vi "ContMeta.vi"(4 "Aux graph ref":refnum<vi>, 6 "CtrlRefsin":T3, 7 "slider refs in":T4, 9 "File Paths":T5={"Local Save Path"=path "\\\\smbhome.uscs.susx.ac.uk\\cv222/Desktop/data", "Newton Save Path"=path "Z:/#Projects/Entanglement/data", "File Name"="test", "LocalSave"=TRUE}, 10 "Compiler Settings":T6={"Python Path"=path "", "Main File"="makesequence.py", "Meta File"="makesequence.py", "Aux File"="makesequence.py", "Pre File"="metascript.txt"}, 11 "ControllerSettingsRef":refnum<vi>) -> ()   [LabVIEW 2019]
uses:
  PulseCompiler/CompilerSettings.ctl
  controls/FilePaths.ctl
  controls/FluoSettings.ctl
  controls/xAOMSettings/XAOMsetting.xctl
  controls/PowerStableSettings.ctl
  PulseControl.ctl
  Compiler/Params.ctl
  controls/ControllerSettings.ctl
  controls/GlobalExp.vi
  Global.lvlib
panel:
  out "calib":bool
  out "Aux Pulse":T1
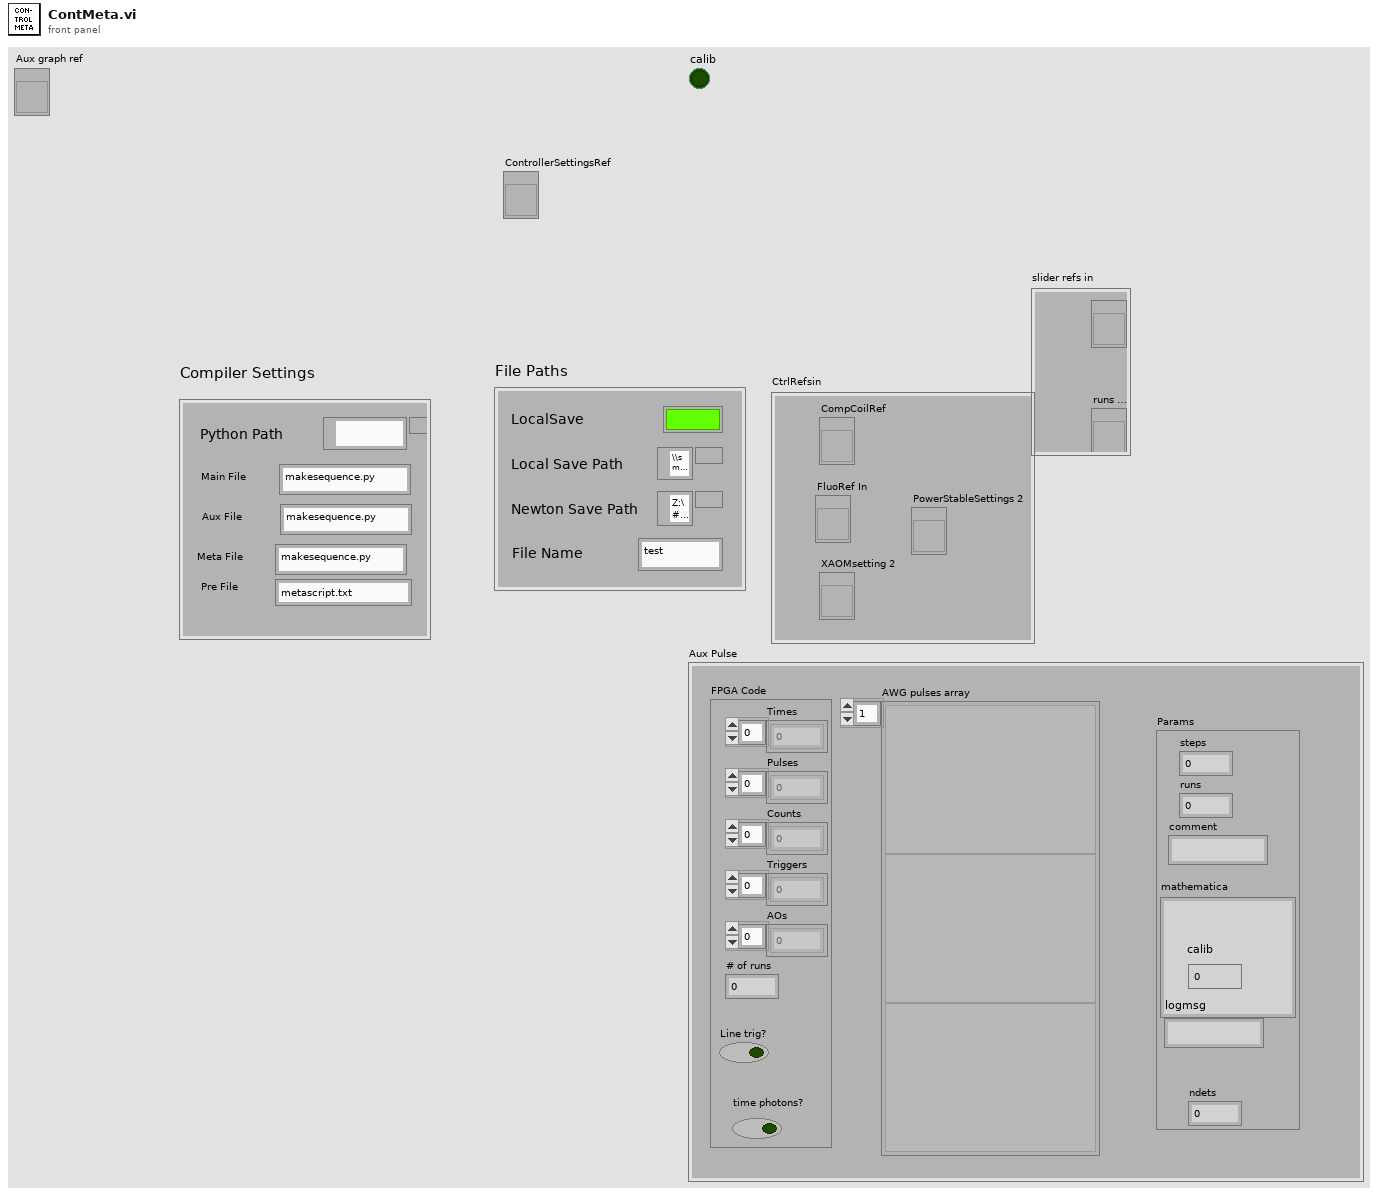
[diagram p1: front panel]
types:
  T1 = typedef "PulseControl.ctl" = cluster{"FPGA Code":cluster{"Times":u32[], "Pulses":u64[], "Counts":u8[], "Triggers":u8[], "AOs":u8[], "# of runs":i32, "Line trig?":bool, "time photons?":bool}, "AWG pulses array":variant[], "Params":T2}
  T2 = typedef "Params.ctl" = cluster{"steps":i16, "runs":i16, "comment":string, "mathematica":string, "calib":i8, "logmsg":string, "ndets":i16}
  T3 = cluster{"CompCoilRef":refnum<vi>, "FluoRef In":refnum<vi>, "XAOMsetting 2":refnum<vi>, "PowerStableSettings 2":refnum<vi>}
  T4 = cluster{"steps slider ref":refnum<vi>, "runs slider ref":refnum<vi>}
  T5 = typedef "FilePaths.ctl" = cluster{"Local Save Path":path, "Newton Save Path":path, "File Name":string, "LocalSave":bool}
  T6 = typedef "CompilerSettings.ctl" = cluster{"Python Path":path, "Main File":string, "Meta File":string, "Aux File":string, "Pre File":string}
  T7 = enum16{"Innit", "Stop", "Idle", "MainRunning", "AuxRunning"}
  T8 = typedef "MasterExpControl.ctl" = cluster{"Main Steps":dbl, "Main Runs":dbl, "ExpStatus":enum16{"Innit", "Stop", "Idle", "MainRunning", "AuxRunning"}, "Main Current Step":dbl, "ExpNum":dbl, "NewData":bool, "date":string, "command":string, "Stop":bool, "Pause":bool, "Mathematica":string, "Main/Meta":bool, "UpdateMath":bool, "Camera":bool, "MetaExpOver":bool, "NextMetaExp":bool}
  T9 = typedef "ControllerSettings.ctl" = cluster{"Aux Sequence":bool, "Camera":bool, "Recrystallize":bool, "Raw graph":bool, "Mean graph":bool, "Calculate probs":bool, "Find fit":bool, "ReX Time [s] :":dbl, "Lock Voltage :":dbl, "Line trig ":bool, "Check Fluo":bool, "Pre Sequence":bool}
  T10 = cluster{"readout":u32[][], "kinetic series data":i32[][][][], "camera dim":cluster{i32, i32, i32, i32}}
  T11 = cluster{"readout out 2":dbl[][], "kinetic series data":i32[][][][], "camera dim":cluster{i32, i32, i32, i32}}
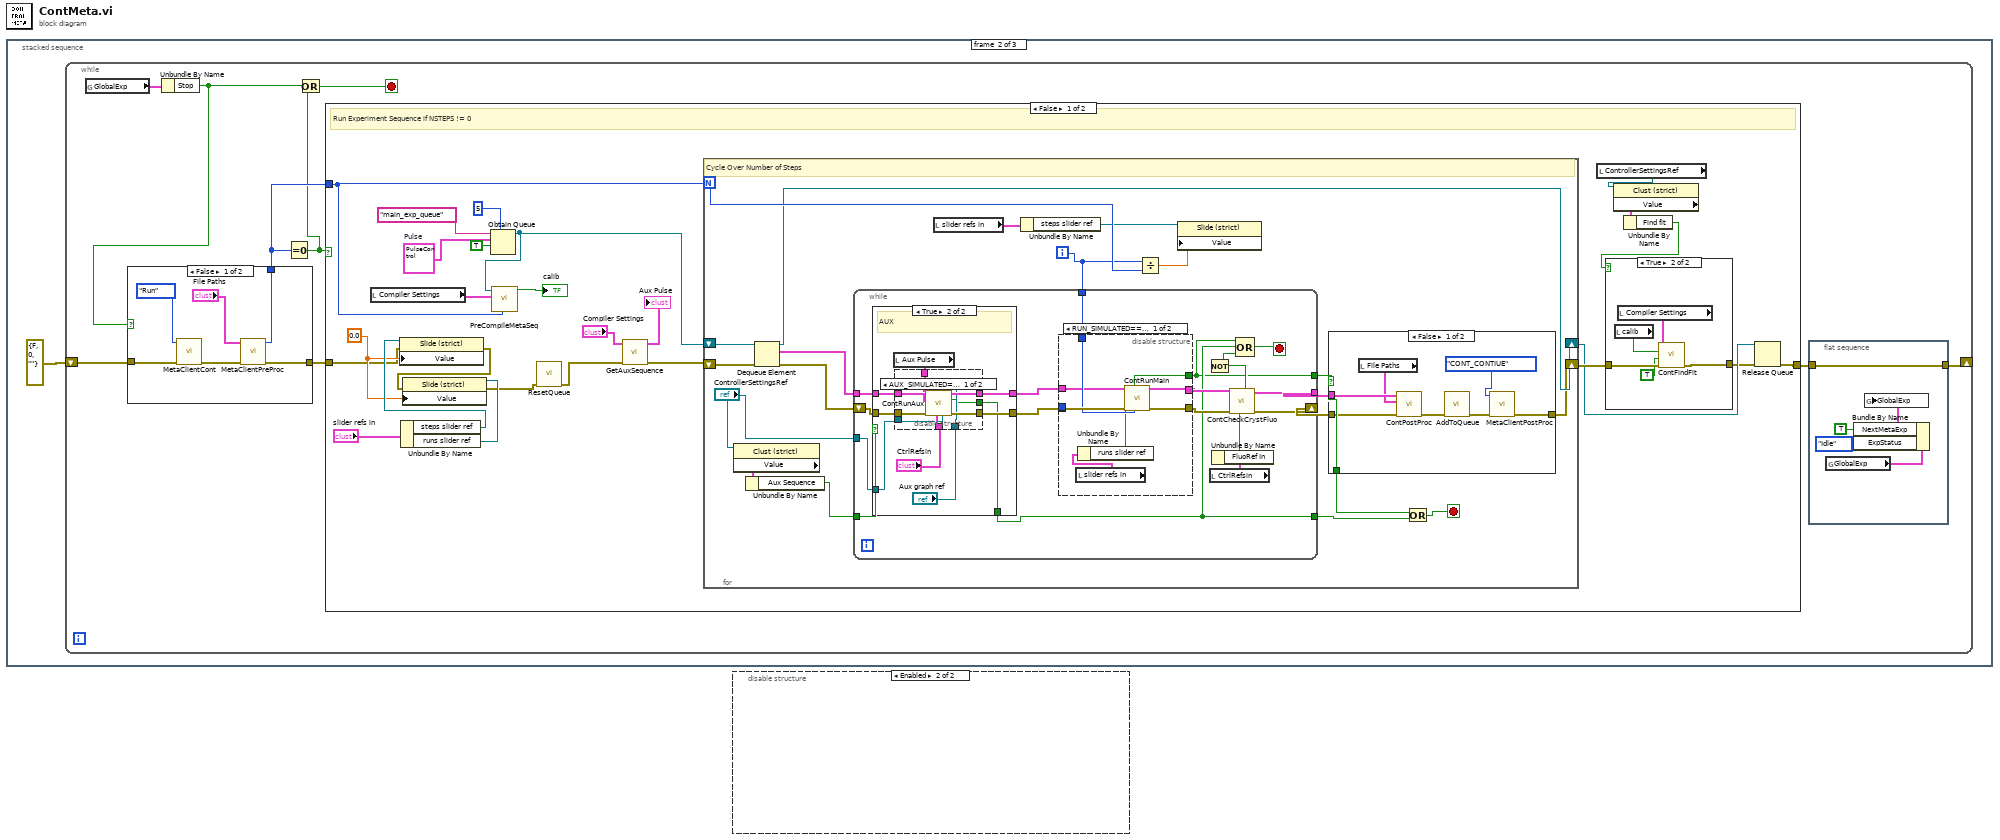
[diagram p0: block diagram]
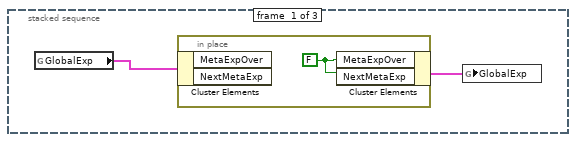
[diagram p2: hidden frame]
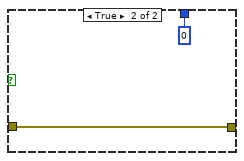
[diagram p3: hidden frame]
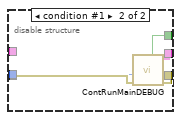
[diagram p5: hidden frame]
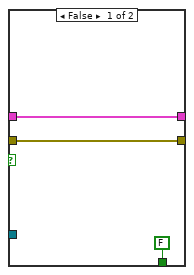
[diagram p6: hidden frame]
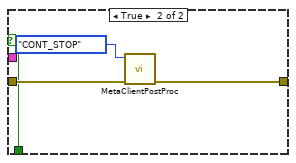
[diagram p8: hidden frame]
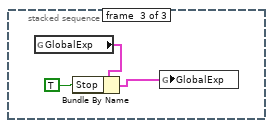
[diagram p10: hidden frame]
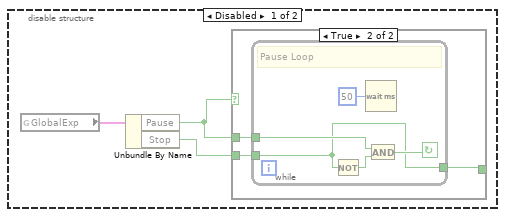
[diagram p11: hidden frame]
diagram:
  n1 = stacked-sequence {
    frame #0 {
      n2 = global read "GlobalExp.vi" "GlobalExp"() -> (w2:T8)
      n3 = in-place {
        w3 = FALSE
        n4 = in-place-cluster #1(w2) -> ()  [unwired: 2 out]
        n5 = in-place-cluster #1("MetaExpOver"=w3, "NextMetaExp"=w3) -> (w1:T8)
      }
      n6 = global write "GlobalExp.vi" "GlobalExp"(w1) -> ()
    }
    frame #1 {
      n7 = while {
        shift-right: [w11] -> _
        shift-left: errorcluster {"status"=FALSE, "code"=0, "source"=""} ("error out") -> [w13]
        stop <- w9 stop-if-true
        n8 = global read "GlobalExp.vi" "GlobalExp"() -> (w6:T8)
        n9 = Unbundle By Name(w6) -> ("Stop"=w8:bool)
        n10 = case shown="False" w8 {
          tunnel: w13 -> [w19 w20]
          tunnel: [w15 w20] -> w12
          tunnel: [w14 0 ("steps")] -> w10
          frame False {
            n11 = call "MetaClientCont.vi"("error in (no error)"=w19, "Action"=enum16{"Run", "Exit"}."Run") -> ("error out"=w17:errorcluster)  [unwired: 8 in, 1 out]
            n12 = call "MetaClientPreProc.vi"("error in (no error)"=w17, "File Paths"="File Paths") -> ("error out"=w15:errorcluster, "steps"=w14:i32)  [unwired: 7 in, 1 out]
          }
          frame True {
          }
        }
        n13 = Equal To 0?(x=w10) -> (x = 0?=w7:bool)
        n14 = Or(x=w8, y=w7) -> (x .or. y?=w9:bool)
        n15 = case shown="False" w7 {
          tunnel: w12 -> [w31 w140]
          tunnel: [w23 w140] -> w5
          tunnel: w10 -> [w36 _]
          frame False {
            w32 = 0.0 ("Value")
            w43 = T1 {"FPGA Code"={"Times"=[], "Pulses"=[], "Counts"=[], "Triggers"=[], "AOs"=[], "# of runs"=0, "Line trig?"=FALSE, "time photons?"=FALSE}, "AWG pulses array"=[], "Params"={"steps"=0, "runs"=0, "comment"="", "mathematica"="", "calib"=0, "logmsg"="", "ndets"=0}}  # Pulse
            # "Run Experiment Sequence if NSTEPS != 0"
            n16 = local read "Compiler Settings"() -> (w41:T6)
            n17 = Unbundle By Name("slider refs in") -> ("steps slider ref"=w33:refnum<vi>, "runs slider ref"=w34:refnum<vi>)
            n18 = property class="Slide (strict)"(reference=w33, error in=w31, "Value"=w32) -> (error out=w30:errorcluster)  [unwired: 1 out]
            n19 = property class="Slide (strict)"(reference=w34, error in=w30, "Value"=w32) -> (error out=w28:errorcluster)  [unwired: 1 out]
            n20 = Obtain Queue(max queue size (-1, unlimited)=5, name (unnamed)="main_exp_queue", element data type=w43, create if not found? (T)=TRUE) -> (queue out=w40:refnum<queue>)  [unwired: 1 in, 2 out]
            n21 = call "PreCompileMetaSeq.vi"("steps"=w36, "Compiler Settings"=w41, "queue in"=w40) -> ("calib"=→"calib":bool)  [unwired: 7 in, 1 out]
            n22 = call "ResetQueue.vi"("error constant"=w28) -> ("error constant 2"=w29:errorcluster)  [unwired: 10 in]
            n23 = call "GetAuxSequence.vi"("error in (no error)"=w29, "Compiler Settings"="Compiler Settings") -> ("error out"=w47:errorcluster, "Aux Pulse"=→"Aux Pulse":T1)  [unwired: 8 in]
            n24 = for {
              N: w36 -> [w71]
              shift-right: [w59] -> w38
              shift-left: w47 -> [w68]
              shift-right: [w60] -> w25
              shift-left: w40 -> [w66]
              i -> [w61]
              stop <- w58 stop-if-true
              # "Cycle Over Number of Steps"
              n25 = property class="Clust (strict)"(reference="ControllerSettingsRef") -> ("Value"=w55:T9)  [unwired: 1 in, 2 out]
              n26 = Unbundle By Name(w55) -> ("Aux Sequence"=w64:bool)
              n27 = Dequeue Element(queue=w66, error in (no error)=w68) -> (queue out=w60:refnum<queue>, element=w65:T1, error out=w67:errorcluster)  [unwired: 1 in, 1 out]
              n28 = while {
                tunnel: [w75] -> w72
                tunnel: w65 -> [w90]
                tunnel: [w83] -> w62
                tunnel: w61 -> [w87]
                tunnel: "ControllerSettingsRef" -> [w85]
                shift-right: [w82] -> w63
                shift-left: w67 -> [w91]
                tunnel: w64 -> [w88]
                tunnel: [w76] -> w56
                stop <- w74 stop-if-true
                n29 = case shown="True" w88 {
                  tunnel: [w107 w117] -> w86
                  tunnel: w91 -> [w108 w116]
                  tunnel: [w108 w115] -> w89
                  tunnel: w90 -> [w107 w112]
                  tunnel: [FALSE ("Aux stopped") w110] -> w76
                  tunnel: w85 -> [_ w109]
                  frame False {
                  }
                  frame True {
                    # "AUX"
                    n30 = local read "Aux Pulse"() -> (w111:T1)
                    n31 = disable-structure shown="AUX_SIMULATED==FALSE, Default" {
                      disable-tunnel: [w126 _] -> w117
                      disable-tunnel: w116 -> [w125 w127]
                      disable-tunnel: [w124 w127] -> w115
                      disable-tunnel: "Aux graph ref" -> [w123 _]
                      disable-tunnel: "CtrlRefsin" -> [w122 _]
                      disable-tunnel: w112 -> [w121 _]
                      disable-tunnel: w111 -> [w120 _]
                      disable-tunnel: [w119 _] -> w110
                      disable-tunnel: w109 -> [w118 _]
                      frame condition #0 (active) {
                        n32 = call "ContRunAux.vi"("ControllerSettingsRef"=w118, "CtrlRefsin"=w122, "Aux chart ref in"=w123, "error in (no error)"=w125, "Aux pulse in"=w120, "Main Pulse In"=w121) -> ("error out"=w124:errorcluster, "Aux stopped"=w119:bool, "Main Pulse Out"=w126:T1)  [unwired: 3 in]
                      }
                      frame condition #1 {
                      }
                    }
                  }
                }
                n33 = disable-structure shown="RUN_SIMULATED==FALSE" {
                  disable-tunnel: [w97 w105] -> w84
                  disable-tunnel: w89 -> [w99 w104]
                  disable-tunnel: [w98 w103] -> w81
                  disable-tunnel: [w96 w101] -> w75
                  disable-tunnel: _ -> [_ w100]
                  disable-tunnel: w87 -> [w95 _]
                  disable-tunnel: w86 -> [w92 _]
                  frame condition #0 (active) {
                    n34 = local read "slider refs in"() -> (w94:T4)
                    n35 = Unbundle By Name(w94) -> ("runs slider ref"=w93:refnum<vi>)
                    n36 = call "ContRunMain.vi"("Step Number"=w95, "error in"=w99, "runs slider ref"=w93, "Main Pulse In"=w92) -> ("error out"=w98:errorcluster, "readout"=w97:T10, "Stop"=w96:bool)  [unwired: 5 in]
                  }
                  frame condition #1 {
                    n37 = call "ContRunMainDEBUG.vi"("error in (no error)"=w104, "step num"=w100) -> ("error out"=w103:errorcluster, "readout"=w105:T11, "Stop"=w101:bool, "runs slider ref"=w102:refnum<vi>)  [unwired: 6 in]
                  }
                }
                n38 = local read "CtrlRefsin"() -> (w78:T3)
                n39 = Unbundle By Name(w78) -> ("FluoRef In"=w77:refnum<vi>)
                n40 = call "ContCheckCrystFluo.vi"("FluoRef In"=w77, "error in (no error)"=w81, "readout"=w84) -> ("error out"=w82:errorcluster, "readout 2"=w83:T10, "restart step?"=w79:bool)  [unwired: 6 in]
                n41 = Not(x=w79) -> (.not. x?=w80:bool)
                n42 = Compound Arithmetic op=OR(w75, w76, w80) -> (w74:bool)
              }
              n43 = local read "slider refs in"() -> (w70:T4)
              n44 = Unbundle By Name(w70) -> ("steps slider ref"=w69:refnum<vi>)
              n45 = Divide(x=w61, y=w71) -> (x/y=w73:dbl)
              n46 = property class="Slide (strict)"(reference=w69, "Value"=w73) -> ()  [unwired: 1 in, 2 out]
              n47 = case shown="False" w72 {
                selector: w72 -> [w133 w136]
                tunnel: w63 -> [w128 w138]
                tunnel: [w135 w137] -> w59
                tunnel: [w133 w136] -> w57
                tunnel: w62 -> [w132 _]
                frame False {
                  n48 = local read "File Paths"() -> (w131:T5)
                  n49 = call "ContPostProc.vi"("Error In"=w128, "File Paths"=w131, "readout"=w132) -> ("error out"=w130:errorcluster)  [unwired: 8 in]
                  n50 = call "AddToQueue.vi"("error constant"=w130) -> ("error constant 2"=w129:errorcluster)  [unwired: 10 in]
                  n51 = call "MetaClientPostProc.vi"("error in (no error)"=w129, "postproc action"=enum16{"CONT_IDLE", "CONT_CONTIUE", "CONT_STOP"}."CONT_CONTIUE") -> ("error out"=w135:errorcluster)  [unwired: 9 in]
                }
                frame True {
                  n52 = call "MetaClientPostProc.vi"("error in (no error)"=w138, "postproc action"=enum16{"CONT_IDLE", "CONT_CONTIUE", "CONT_STOP"}."CONT_STOP") -> ("error out"=w137:errorcluster)  [unwired: 9 in]
                }
              }
              n53 = Or(x=w57, y=w56) -> (x .or. y?=w58:bool)
            }
            n54 = local read "ControllerSettingsRef"() -> (w26:refnum<vi>)
            n55 = property class="Clust (strict)"(reference=w26) -> ("Value"=w27:T9)  [unwired: 1 in, 2 out]
            n56 = Unbundle By Name(w27) -> ("Find fit"=w37:bool)
            n57 = case shown="True" w37 {
              tunnel: w38 -> [w48 w52]
              tunnel: [w48 w51] -> w24
              frame False {
              }
              frame True {
                n58 = local read "calib"() -> (w49:bool)
                n59 = local read "Compiler Settings"() -> (w53:T6)
                n60 = call "ContFindFit.vi"("error in (no error)"=w52, "GenImage"=TRUE, "update"=w49, "Compiler Settings"=w53) -> ("error out"=w51:errorcluster)  [unwired: 7 in]
              }
            }
            n61 = Release Queue(queue=w25, error in (no error)=w24) -> (error out=w23:errorcluster)  [unwired: 1 in, 2 out]
          }
          frame True {
          }
        }
        n62 = flat-sequence {
          tunnel: [w141] -> w11
          tunnel: w5 -> [w141]
          frame #0 {
            n63 = global read "GlobalExp.vi" "GlobalExp"() -> (w144:T8)
            n64 = Bundle By Name(cluster=w144, "NextMetaExp"=TRUE ("MetaExpOver"), "ExpStatus"=T7."Idle") -> (w145:T8)
            n65 = global write "GlobalExp.vi" "GlobalExp"(w145) -> ()
          }
        }
      }
    }
    frame #2 {
      n66 = global read "GlobalExp.vi" "GlobalExp"() -> (w148:T8)
      n67 = Bundle By Name(cluster=w148, "Stop"=TRUE) -> (w147:T8)
      n68 = global write "GlobalExp.vi" "GlobalExp"(w147) -> ()
    }
  }
  n69 = disable-structure shown="Enabled" {
    frame Disabled {
      n70 = global read "GlobalExp.vi" "GlobalExp"() -> (w151:T8)
      n71 = Unbundle By Name(w151) -> ("Pause"=w150:bool, "Stop"=w149:bool)
      n72 = case shown="True" w150 {
        tunnel: w150 -> [_ w155]
        tunnel: w149 -> [w152 w154]
        tunnel: [w152 w153] -> _
        frame False {
        }
        frame True {
          n73 = while {
            tunnel: w155 -> [w157]
            tunnel: w154 -> [w156]
            tunnel: [w156] -> w153
            stop <- w159 continue-if-true
            # "Pause Loop"
            n74 = Not(x=w156) -> (.not. x?=w158:bool)
            n75 = Wait (ms)(milliseconds to wait=u32 50) -> ()  [unwired: 1 out]
            n76 = And(x=w157, y=w158) -> (x .and. y?=w159:bool)
          }
        }
      }
    }
    frame Enabled {
    }
  }
